vi "create_save_parameters.vi"(6 "timestamp":string, 8 "Measurement settings":T1={"Minimum LED current (A)"=300.0, "Maximum LED Current (A)"=900.0, "Number of LED currents in sweep"=5, "LED current sweep mode"=8, "LED current sweep direction"=8, "LED settling delay (ms)"=500, "Solar cell measurement mode"=0, "Minimum JV voltage (V)"=1.0, "Maximum JV voltage (V)"=1.0, "JV voltage step (V)"=8.0, "JV sweep direction"=1, "Dual JV sweep"=50, "Current range"=4, "Voltage range"=4, "Integration time (NPLC)"=1, "Auto settling delay"=0, "Settling delay (ms)"=0.0, "Enable display"=0} {"Voltage range" items=["Auto", "200 mV", "2.1 V", "21 V", "210 V"]; "Enable display" items=["False", "True"]; "Auto settling delay" items=["False", "True"]; "Settling delay (ms)" min=0.2 max=999999.9; "Integration time (NPLC)" items=["0.01", "0.1", "1", "10"]; "Current range" items=["Auto", "1 uA", "10 uA", "100 uA", "1 mA", "10 mA", "100 mA", "1 A"]; "Dual JV sweep" items=["False", "True"]; "JV sweep direction" items=["Ascending", "Descending"]; "JV voltage step (V)" min=0.0001 max=5.0 step=0.0001; "Solar cell measurement mode" items=["J-V", "Voc", "Jsc"]; "LED current sweep direction" items=["Ascending", "Descending"]; "LED current sweep mode" items=["Linear", "Logarithmic"]; "Maximum LED Current (A)" min=0.0 max=0.7 step=0.001 format="%#.3f"; "Minimum LED current (A)" min=0.0 max=0.7 step=0.001 format="%#.3f"}, 9 "Device details":T2={"Device label"="", "Pixel"=enum."1", "Area (cm^2)"=0.0}, 10 "Experiment Title":string, 11 "Username":string) -> (2 "settings path":path, 3 "experiment folder":path)   [LabVIEW 2018]
uses:
  typedefs/device_details.ctl
  typedefs/measurement_settings.ctl
  <vilib>/Utility/file.llb/Write Delimited Spreadsheet (string).vi
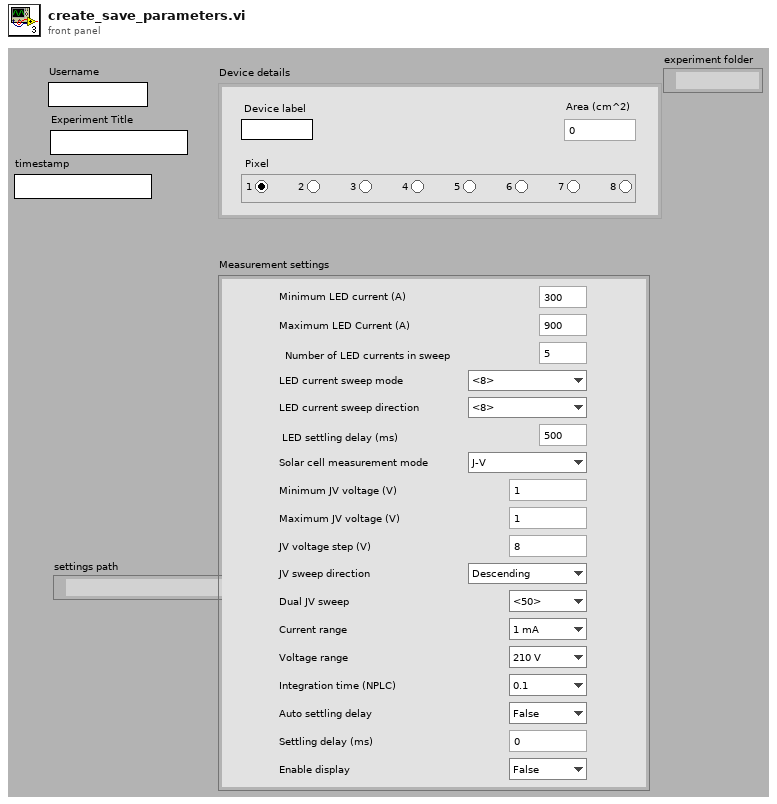
[diagram p1: front panel]
types:
  T1 = typedef "measurement_settings.ctl" = cluster{"Minimum LED current (A)":dbl, "Maximum LED Current (A)":dbl, "Number of LED currents in sweep":u32, "LED current sweep mode":u16, "LED current sweep direction":u16, "LED settling delay (ms)":u32, "Solar cell measurement mode":u16, "Minimum JV voltage (V)":dbl, "Maximum JV voltage (V)":dbl, "JV voltage step (V)":dbl, "JV sweep direction":u16, "Dual JV sweep":u16, "Current range":u16, "Voltage range":u16, "Integration time (NPLC)":u16, "Auto settling delay":u16, "Settling delay (ms)":dbl, "Enable display":u16}
  T2 = typedef "device_details.ctl" = cluster{"Device label":string, "Pixel":enum32{"No Selection", "1", "2", "3", "4", "5", "6", "7", "8"}, "Area (cm^2)":dbl}
  T3 = enum32{"No Selection", "1", "2", "3", "4", "5", "6", "7", "8"}
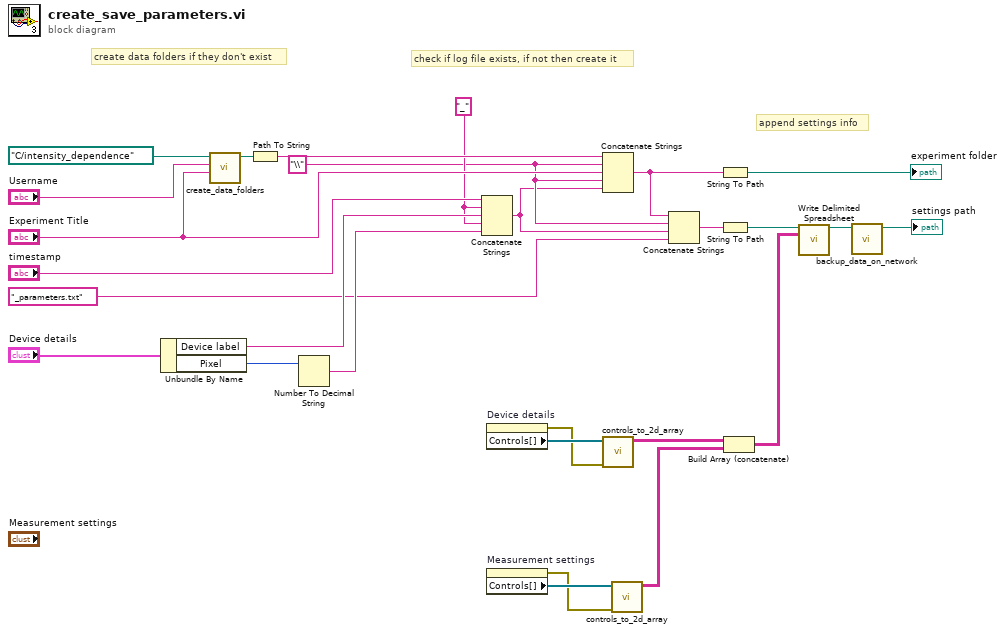
[diagram p0: block diagram]
diagram:
  w15 = "_"
  w12 = "\\"
  # "append settings info"
  # "create data folders if they don't exist"
  # "check if log file exists, if not then create it"
  n1 = Unbundle By Name("Device details") -> ("Device label"=w16:string, "Pixel"=w22:T3)
  n2 = call "create_data_folders.vi"("Experiment Title"="Experiment Title", "Username"="Username", "Folderpath on C:"=path "C:/intensity_dependence") -> ("Folderpath on C: out"=w27:path)  [unwired: 8 in]
  n3 = Path To String(path=w27) -> (string=w26:string)
  n4 = Number To Decimal String(number=w22) -> (decimal integer string=w14:string)  [unwired: 1 in]
  n5 = Concatenate Strings("timestamp", w15, w16, w15, w14) -> (w11:string)
  n6 = property on="Device details" class="Clust (strict)"() -> (error out=w4:errorcluster, "Controls[]"=w5:refnum<vi>[])  [unwired: 2 in, 1 out]
  n7 = property on="Measurement settings" class="Clust (strict)"() -> (error out=w6:errorcluster, "Controls[]"=w7:refnum<vi>[])  [unwired: 2 in, 1 out]
  n8 = Concatenate Strings(w26, w12, "Experiment Title", w12, w11) -> (w13:string)
  n9 = call "controls_to_2d_array.vi"("error in (no error)"=w4, "Controls[]"=w5) -> ("Array"=w3:string[][])  [unwired: 9 in]
  n10 = call "controls_to_2d_array.vi"("error in (no error)"=w6, "Controls[]"=w7) -> ("Array"=w2:string[][])  [unwired: 9 in]
  n11 = Concatenate Strings(w13, w12, w11, "_parameters.txt") -> (w9:string)
  n12 = String To Path(string=w13) -> (path=→"experiment folder":path)
  n13 = String To Path(string=w9) -> (path=w8:path)
  n14 = Build Array (concatenate)(w3, w2) -> (w1:string[][])
  n15 = call-poly <vilib>:"Write Delimited Spreadsheet.vi"("file path (dialog if empty)"=w8, "2D data"=w1) -> ("new file path (Not A Path if cancelled)"=w21:path)  [unwired: 12 in, 1 out]
  n16 = call "backup_data_on_network.vi"("Filepath in"=w21) -> ("Filepath out"=→"settings path":path)  [unwired: 10 in]
